vi "get_voltage_limits.vi"(8 "error in (no error)":errorcluster, 11 "PZT in":refnum<class "PZT.lvclass">) -> (0 "error out":errorcluster, 1 "voltage_furthest (bits)":i16, 2 "voltage_closest (bits)":i16, 3 "PZT out":refnum<class "PZT.lvclass">)   [LabVIEW 2020, in "PZT.lvclass"]
uses:
  PZT.lvclass
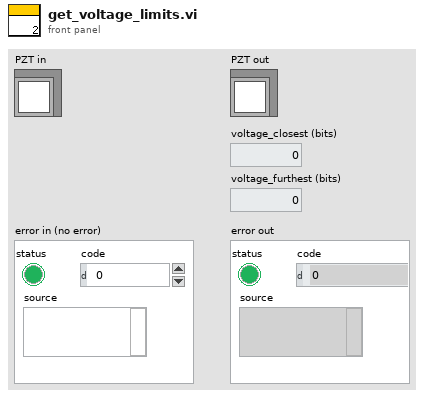
[diagram p1: front panel]
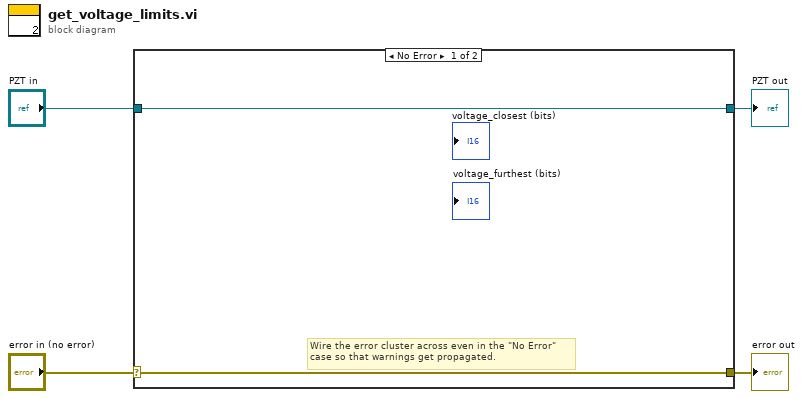
[diagram p0: block diagram]
diagram:
  n1 = case shown="No Error" "error in (no error)" {
    selector: "error in (no error)" -> [w5 w8]
    tunnel: [w5 w8] -> w3
    tunnel: [w6 w7] -> w1
    tunnel: "PZT in" -> [w6 w7]
    frame No Error {
      # "Wire the error cluster across even in the \"No Error\"\ncase so that warnings get propagated."
    }
    frame Error {
    }
  }
  "error out" <- w3
  "PZT out" <- w1
